vi "Ctor.vi"(8 "error in (no error)":errorcluster, 11 "Width (0)":i32) -> (0 "error out":errorcluster, 3 "TermLine out":refnum<class "TermLine.lvclass">)   [LabVIEW 2020, in "Terminal.lvlib" / "TermLine.lvclass"]
uses:
  TermLine.lvclass
  Ref Data.ctl
  Term Char.ctl
  TermLine.lvclass/TermLine.ctl
  Terminal.lvlib
  Text Attributes.ctl
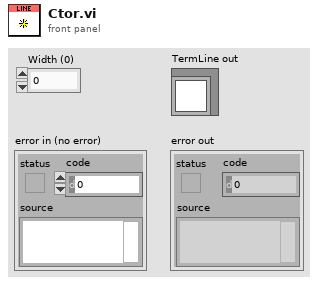
[diagram p1: front panel]
types:
  T1 = typedef "Terminal.lvlib/Term Char.ctl" = cluster{"Char":string, "Attributes":T2}
  T2 = typedef "Terminal.lvlib/Text Attributes.ctl" = cluster{"FG":u32, "BG":u32, "Bold":bool, "Italic":bool, "Underline":bool, "Strike":bool, "Inverse":bool}
  T3 = typedef "Terminal.lvlib/TermLine.lvclass/Ref Data.ctl" = cluster{"Chars":T1[], "Width":i32}
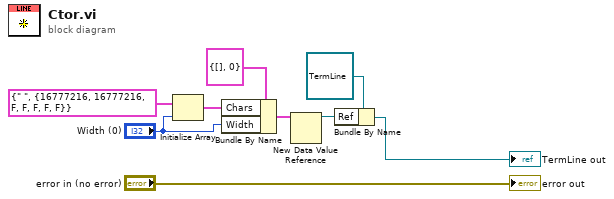
[diagram p0: block diagram]
diagram:
  n1 = Initialize Array(T1 {"Char"=" ", "Attributes"={"FG"=16777216, "BG"=16777216, "Bold"=FALSE, "Italic"=FALSE, "Underline"=FALSE, "Strike"=FALSE, "Inverse"=FALSE}} ("Term Char"), "Width (0)") -> (w5:T1[])
  n2 = Bundle By Name(cluster=T3 {"Chars"=[], "Width"=0} ("Ref Data"), "Chars"=w5, "Width"="Width (0)") -> (w3:T3)
  n3 = New Data Value Reference(data value=w3) -> (data value reference=w1:refnum<data-value>)  [unwired: 1 in, 1 out]
  n4 = Bundle By Name(cluster=refnum<class "TermLine.lvclass"> refnum ("TermLine in"), "Ref"=w1) -> (→"TermLine out":refnum<class "TermLine.lvclass">)
  "error out" <- "error in (no error)"
